vi "Main_SAIDD.vi"() -> ()   [LabVIEW 2019]
uses:
  <extravilib>/ChannelInstances/Tag-bool/Write With Abort.vi
  <extravilib>/ChannelInstances/Tag-bool/Read With Abort.vi
  <vilib>/myRIO/Common/Instrument Driver Framework/myRIO v1.0/UART/vis/myRIO v1.0 Close UART.vi
  <extravilib>/ChannelInstances/Tag-bool/Instantiate.vi
  <vilib>/Utility/error.llb/Error Cluster From Error Code.vi
  <vilib>/myRIO/Common/Instrument Driver Framework/myRIO v1.0/PWM/vis/myRIO v1.0 Write PWM.vi
  <extravilib>/ChannelInstances/Tag-bool/Endpoint.vi
  <extravilib>/ChannelInstances/Tag-bool/EndpointRead.vi
  <vilib>/myRIO/Common/Instrument Driver Framework/Utilities/vis/FPGA Ref Manager.vi
  <vilib>/myRIO/Common/Instrument Driver Framework/myRIO v1.0/myRIO v1.0 Reset FPGA.vi
  <vilib>/myRIO/Common/Instrument Driver Framework/myRIO v1.0/IRQ/vis/myRIO v1.0 IRQ Info FGV.vi
  <vilib>/myRIO/Common/Instrument Driver Framework/myRIO v1.0/IRQ/vis/myRIO v1.0 Timer IRQ Info FGV.vi
  <vilib>/myRIO/Common/Instrument Driver Framework/myRIO v1.0/IRQ/vis/myRIO v1.0 ISR Agent.vi
  <vilib>/myRIO/Instrument Drivers/Utilities/vis/Reset Index.vi
  <vilib>/myRIO/Common/Instrument Driver Framework/myRIO v1.0/Resource Manager/vis/myRIO v1.0 Block Write Resource Manager.vi
  <extravilib>/ChannelInstances/Tag-bool.lvlib
  <vilib>/myRIO/Instrument Drivers/Onboard IO/DIO/DIO.lvlib
  <vilib>/myRIO/Instrument Drivers/Onboard IO/PWM/PWM.lvlib
  <vilib>/myRIO/Instrument Drivers/Utilities/Utilities.lvlib
panel:
  out "Distance [cm]":dbl
  in  "Antal iterationer pr. stepper":i32=800
  in  "Stop":bool
  out "Measured current":dbl
  out "Ammeter measurement":dbl(graph)
  out "Duty Cycle":dbl
  out "Mean 200":dbl format="%0.2f"
  out "Battery left (%)":dbl
  in  "Drill - Frequency [Hz]":dbl=200.0
  in  "Stepper frekvens ned":dbl=120.0
  in  "Ingen modstand ned upper threshold":dbl=2750.0
  out "ALL TOP":bool
  out "ALL BOTTOM":bool
  in  "Resistance - Threshold Upper":dbl=3175.0
  in  "Resistance Threshold Lower":dbl=2975.0
  out "Process":T1(ring)
  in  "State":T1(ring)
  out "Image":T2(plugin-control)
  in  "high cutoff freq: fh":dbl=900.0
  in  "Radius":dbl=0.002 format="%#_13g"
  in  "Filter?":bool=TRUE
  out "RollDetection - Alarm":bool
  out "Data output (A3 GPS)":string[](array[string])
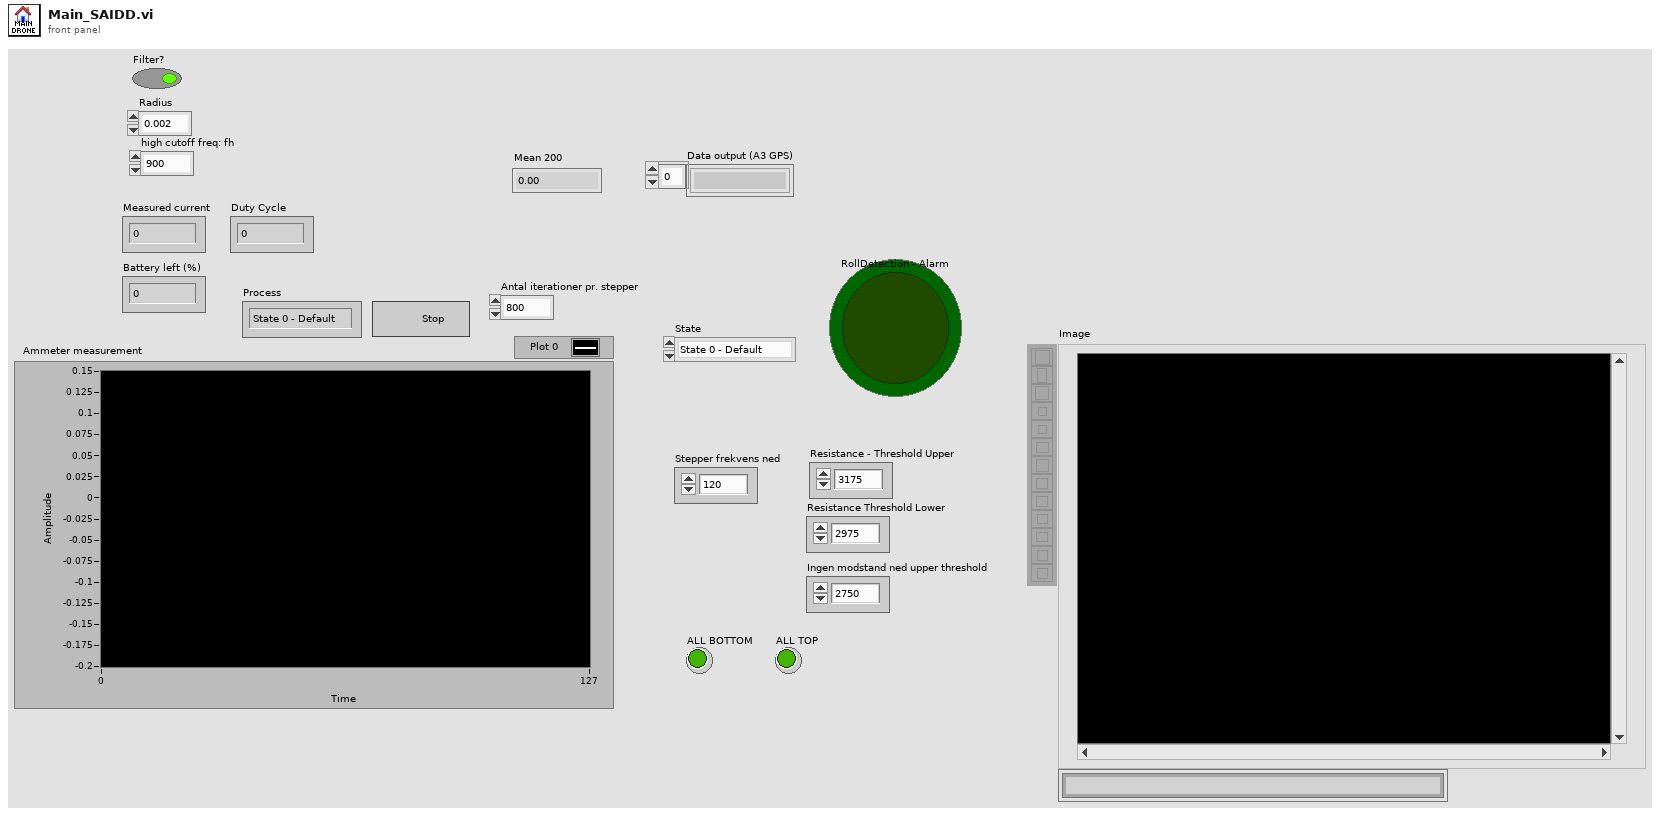
[diagram p1: front panel]
types:
  T1 = enum16{"State 0 - Default", "State 1 - Go down", "State 2 - Go up", "State 3 - Triangle Wobble"}
  T2 = typedef "IMAQ Image.ctl" = refnum<image>
  T3 = typedef "DIO.lvlib/DIO Reference.ctl" = cluster{"myRIO Reference":T4, "DIO Channels List":T8}
  T4 = typedef "myRIO Generic Hardware Reference.ctl" = cluster{"myRIO Model":T5, "myRIO Hardware Reference":T6}
  T5 = typedef "Hardware Version Enum.ctl" = enum16{"Unknown", "myRIO-1900", "myRIO-1950", "roboRIO", "NI ELVIS RIO CM", "ELVIS III"}
  T6 = typedef "myRIO v1.0 Reference.ctl" = cluster{"Generic FPGA Reference":T7, "Allow multiple opens":bool}
  T7 = typedef "Generic FPGA Reference.ctl" = refnum<k20>
  T8 = typedef "DIO Channels List.ctl" = T9[]
  T9 = typedef "DIO Channels Enum.ctl" = enum16{"Not Connected", "C/DIO0", "C/DIO1", "C/DIO2", "C/DIO3", "C/DIO4", "C/DIO5", "C/DIO6", "C/DIO7", "A/DIO0", "A/DIO1", "A/DIO2", "A/DIO3", "A/DIO4", "A/DIO5", "A/DIO6", "A/DIO7", "A/DIO8", "A/DIO9", "A/DIO10", "A/DIO11", "A/DIO12", "A/DIO13", "A/DIO14", "A/DIO15", "A/DIO16", "A/DIO17", "A/DIO18", "A/DIO19", "B/DIO0", "B/DIO1", "B/DIO2", "B/DIO3", "B/DIO4", "B/DIO5", "B/DIO6", "B/DIO7", "B/DIO8", "B/DIO9", "B/DIO10", "B/DIO11", "B/DIO12", "B/DIO13", "B/DIO14", "B/DIO15", "B/DIO16", "B/DIO17", "B/DIO18", "B/DIO19", "LED0", "LED1", "LED2", "LED3", "Button0", "DIO/DIO0", "DIO/DIO1", "DIO/DIO2", "DIO/DIO3", "DIO/DIO4", "DIO/DIO5", "DIO/DIO6", "DIO/DIO7", "DIO/DIO8", "DIO/DIO9", "SPI/CS0", "SPI/CS1", "SPI/CS2", "SPI/CS3", "LED RADIO (Green)", "LED RADIO (Red)", "LED COMM (Green)", "LED COMM (Red)", "LED MODE (Green)", "LED MODE (Red)"}
  T10 = typedef "PWM.lvlib/PWM Reference.ctl" = cluster{"myRIO Reference":T4, "PWM Channels Enum":T11, "PWM Configuration":T12}
  T11 = typedef "PWM Channels Enum.ctl" = enum16{"Not Connected", "C/PWM0", "C/PWM1", "A/PWM0", "A/PWM1", "A/PWM2", "A/PWM3", "A/PWM4", "A/PWM5", "A/PWM6", "A/PWM7", "A/PWM8", "A/PWM9", "A/PWM10", "A/PWM11", "A/PWM12", "A/PWM13", "A/PWM14", "A/PWM15", "A/PWM16", "A/PWM17", "A/PWM18", "A/PWM19", "B/PWM0", "B/PWM1", "B/PWM2", "B/PWM3", "B/PWM4", "B/PWM5", "B/PWM6", "B/PWM7", "B/PWM8", "B/PWM9", "B/PWM10", "B/PWM11", "B/PWM12", "B/PWM13", "B/PWM14", "B/PWM15", "B/PWM16", "B/PWM17", "B/PWM18", "B/PWM19", "PWM/PWM0", "PWM/PWM1", "PWM/PWM2", "PWM/PWM3", "PWM/PWM4", "PWM/PWM5", "PWM/PWM6", "PWM/PWM7", "PWM/PWM8", "PWM/PWM9"}
  T12 = typedef "PWM.lvlib/PWM Configuration.ctl" = cluster{"Frequency":dbl, "Duty Cycle":dbl}
  T13 = typedef "Accelerometer.lvlib/Accelerometer Reference.ctl" = cluster{"myRIO Reference":T4, "Accelerometer Channels List":T14, "LSB Weight":dbl}
  T14 = typedef "Accelerometer Channels List.ctl" = T15[]
  T15 = typedef "Accelerometer Channels Enum.ctl" = enum16{"Not Connected", "X-Axis", "Y-Axis", "Z-Axis"}
  T16 = typedef "AI.lvlib/AI Reference.ctl" = cluster{"myRIO Reference":T4, "AI Channels List":T17, "AI Scaling Constants List":T19}
  T17 = typedef "AI Channels List.ctl" = T18[]
  T18 = typedef "AI Channels Enum.ctl" = enum16{"Not Connected", "AudioIn/Left", "AudioIn/Right", "C/AI0", "C/AI1", "A/AI0", "A/AI1", "A/AI2", "A/AI3", "A/AI4", "A/AI5", "A/AI6", "A/AI7", "B/AI0", "B/AI1", "B/AI2", "B/AI3", "B/AI4", "B/AI5", "B/AI6", "B/AI7", "AI/AI0", "AI/AI1", "AI/AI2", "AI/AI3", "A/AI0 (DIFF)", "A/AI1 (DIFF)", "A/AI2 (DIFF)", "A/AI3 (DIFF)", "B/AI0 (DIFF)", "B/AI1 (DIFF)", "B/AI2 (DIFF)", "B/AI3 (DIFF)"}
  T19 = typedef "Analog Scaling Constants List.ctl" = T20[]
  T20 = typedef "Analog Scaling Constants.ctl" = cluster{"LSB Weight (Volts)":dbl, "Offset (Volts)":dbl, "Signed?":bool}
  T21 = typedef "SPI.lvlib/SPI Reference.ctl" = cluster{"myRIO Reference":T4, "SPI Channels Enum":T22, "SPI Configuration":T23}
  T22 = typedef "SPI Channels Enum.ctl" = enum16{"Not Connected", "A/SPI", "B/SPI", "SPI/SPI"}
  T23 = typedef "SPI.lvlib/SPI Configuration.ctl" = cluster{"Frequency [Hz]":dbl, "Clock Phase":T24, "Clock Polarity":T25, "Data Direction":T26, "Frame Length":T27}
  T24 = typedef "SPI Clock Phase.ctl" = enum8{"Leading", "Trailing"}
  T25 = typedef "SPI Clock Polarity.ctl" = enum8{"Low", "High"}
  T26 = typedef "SPI Data Direction.ctl" = enum8{"Most significant bit first", "Least significant bit first"}
  T27 = typedef "SPI Frame Length.ctl" = u8
  T28 = cluster{"B/DIO0 - Stepper Direction":T3, "B/DIO1 - Stepper1 Enable":T3, "B/DIO2 - Stepper2 Enable":T3, "B/DIO3 - Stepper3 Enable":T3, "B/DIO4 - Endstop Stepper1 Top":T3, "B/DIO11 - Endstop Stepper1 Bund":T3, "B/DIO12 - Endstop Stepper2 Top":T3, "B/DIO13 - Endstop Stepper2 Bund":T3, "B/DIO14 - Endstop Stepper3 Top":T3, "B/DIO15 - Endstop Stepper3 Bund":T3, "A/DIO0 - Cooler":T3, "A/DIO1 - Beacon drop (dio1)":T3, "A/DIO2 - Beacon drop (dio0)":T3, "A/DIO3 - QuickRelease (dio1)":T3, "A/DIO4 - QuickRelease (dio0)":T3, "A/DIO11 - LiDAR SPI CS":T3, "B/PWM0 - Stepper":T10, "B/PWM1 - Drill":T10, "A/PWM0 - Servo_Roll":T10, "A/PWM1 - Servo_Yaw":T10, "Acc. X-axis":T13, "Acc. Y-axis":T13, "B/AI0 - Beacon Drop S1 - F3":T16, "A/AI1 - Stepper Dir S3 - F4":T16, "B/AI2 - Stepper Throttle S4 - F5":T16, "B/AI3 - Drill Throttle S6 - F6":T16, "B/AI0 - Drop Drill S8 - F8":T16, "A/AI1 - Beacon Wiper":T16, "A/AI2 - QuickRelease Wiper":T16, "A/AI3 - Drill Current":T16, "A/SPI - LiDAR":T21, "B/UART - XBee":refnum<visa-resource-name>, "A/UART - A3 GPS":refnum<visa-resource-name>, "RIO Flashing LEDs":T3}
  T29 = typedef "Tag-bool.lvlib/))Channel.ctl" = refnum<queue>
  T30 = typedef "IMAQdx.ctl" = refnum<k21>
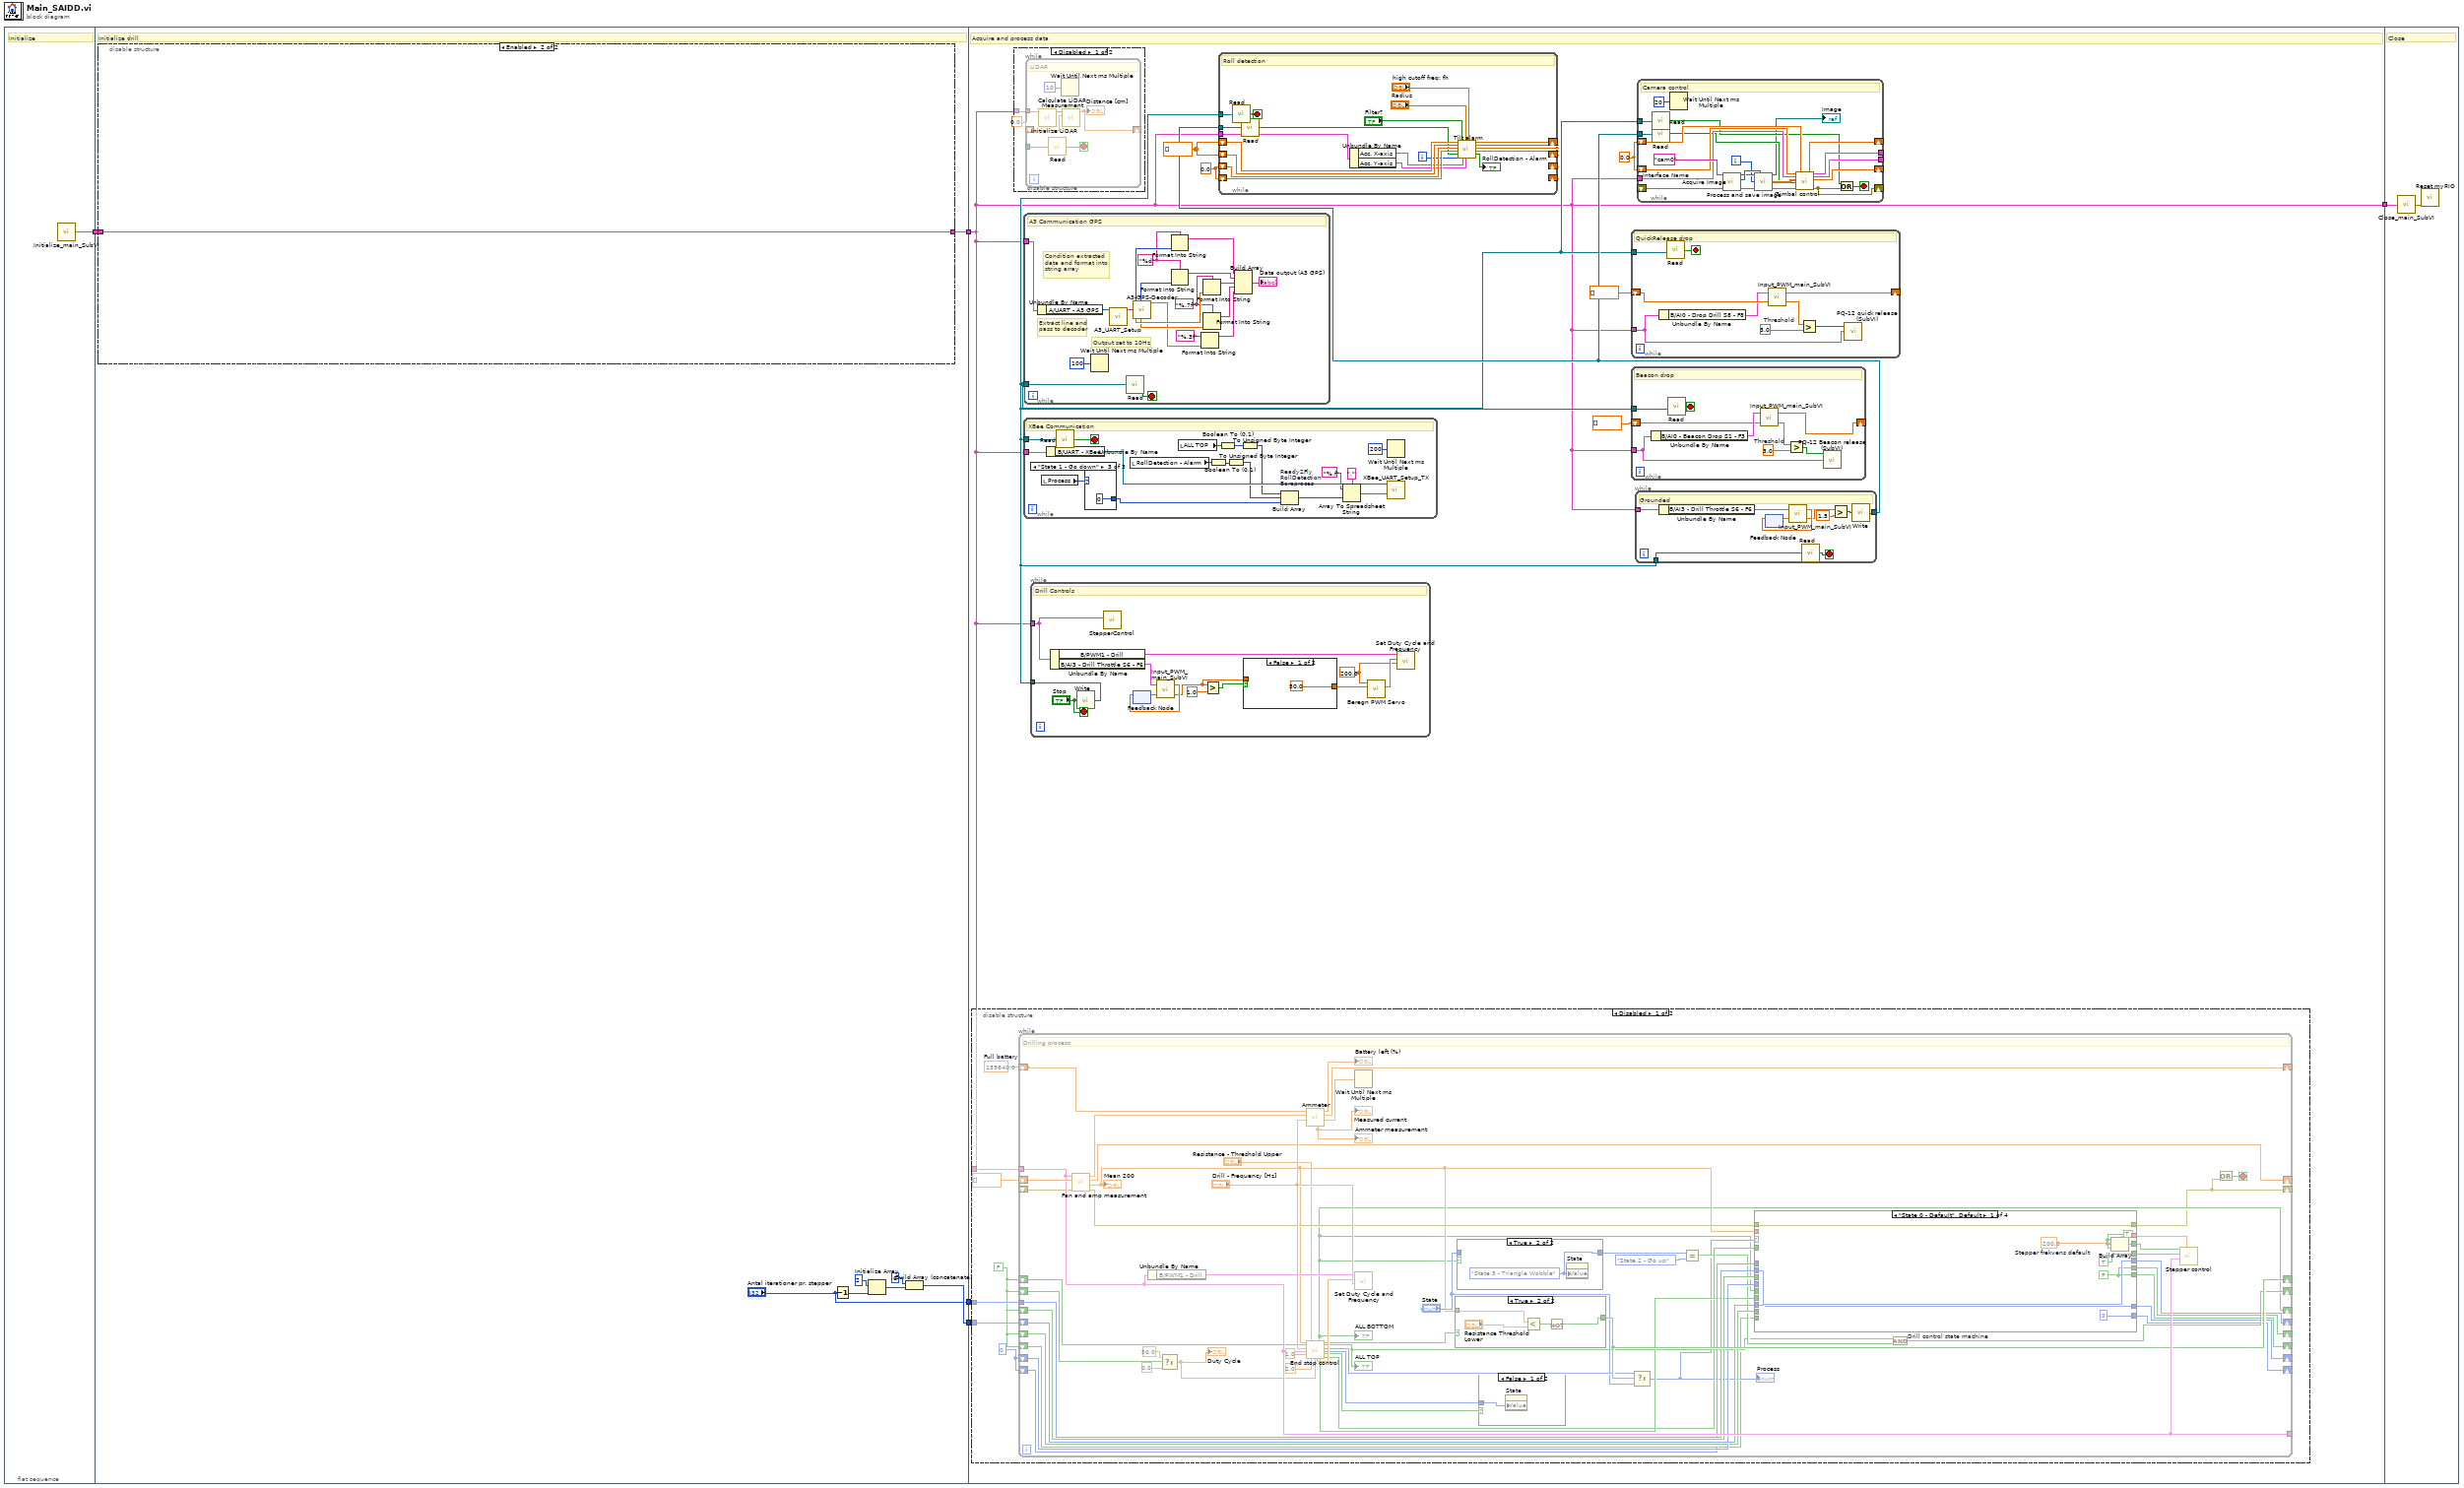
[diagram p0: block diagram]
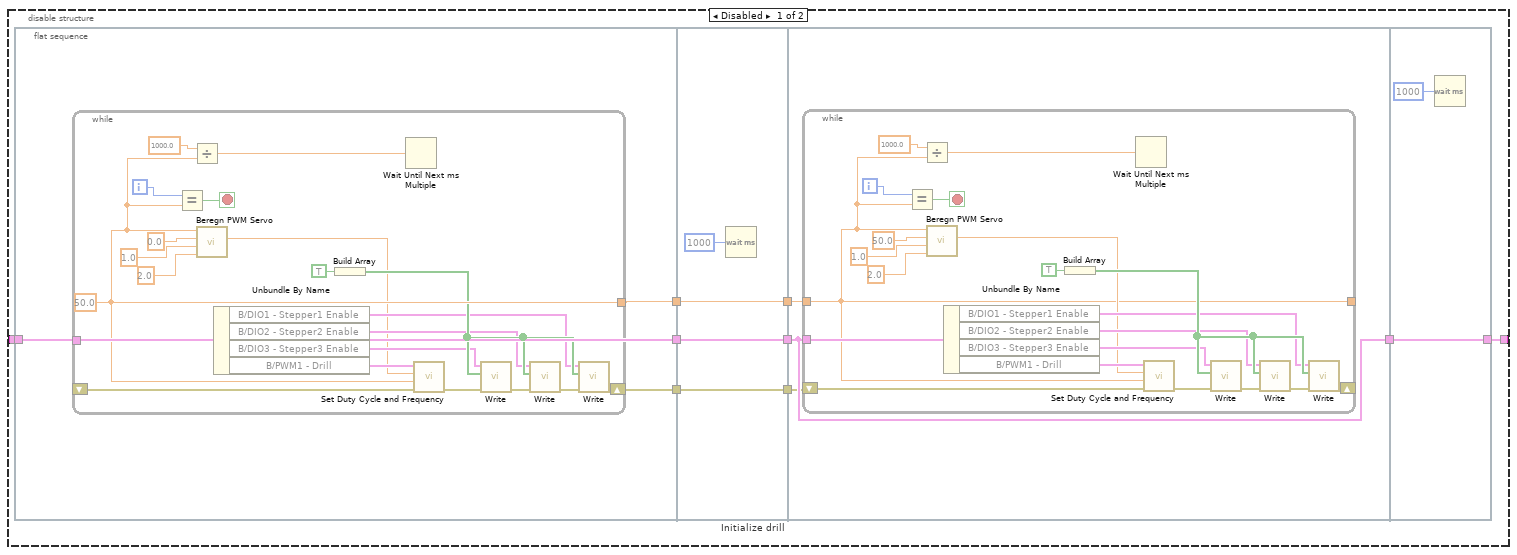
[diagram p2: hidden frame]
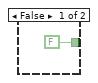
[diagram p5: hidden frame]
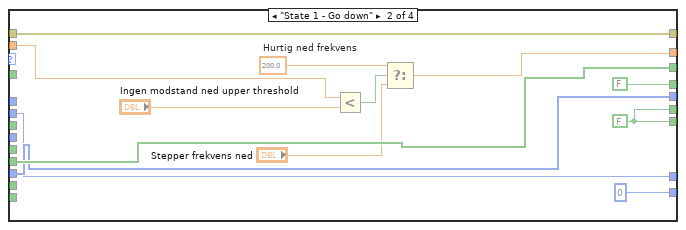
[diagram p6: hidden frame]
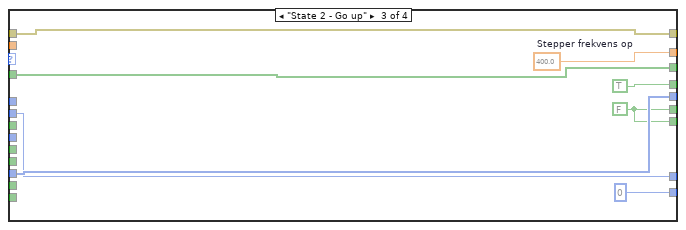
[diagram p7: hidden frame]
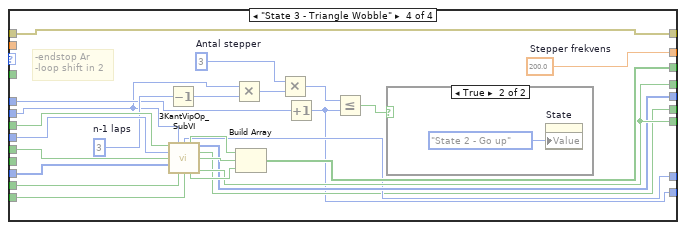
[diagram p8: hidden frame]
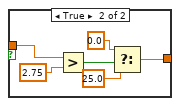
[diagram p11: hidden frame]
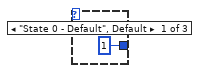
[diagram p13: hidden frame]
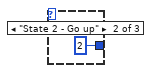
[diagram p14: hidden frame]
diagram:
  n1 = flat-sequence {
    tunnel: [w6] -> w4
    tunnel: w4 -> [w14]
    tunnel: [w13] -> w3
    tunnel: ["Antal iterationer pr. stepper"] -> w2
    tunnel: [w8] -> w1
    tunnel: w3 -> [w79]
    tunnel: [w79] -> w5
    tunnel: w2 -> [w83]
    tunnel: w1 -> [w82]
    tunnel: w5 -> [w357]
    frame #0 {
      # "Initialize"
      n2 = call "Initialize_main_SubVI.vi"() -> ("output cluster"=w6:T28)
    }
    frame #1 {
      # "Initialize drill"
      n3 = disable-structure shown="Enabled" {
        disable-tunnel: w14 -> [w16 w78]
        disable-tunnel: [w15 w78] -> w13
        frame Disabled {
          n4 = flat-sequence "Initialize drill" {
            tunnel: w16 -> [w24]
            tunnel: [w24] -> w23
            tunnel: [w26] -> w22
            tunnel: [w25] -> w21
            tunnel: w23 -> [w51]
            tunnel: [w51] -> w20
            tunnel: [w49] -> w19
            tunnel: w22 -> [w49]
            tunnel: [w48] -> w18
            tunnel: w21 -> [w48]
            tunnel: w20 -> [w54]
            tunnel: [w54] -> w17
            tunnel: w19 -> [w53]
            tunnel: w18 -> [w52]
            tunnel: [w77] -> w15
            tunnel: w17 -> [w77]
            frame #0 {
              n5 = while {
                tunnel: [w41] -> w26
                shift-right: [w33] -> w25
                shift-left: _ -> [w44]
                tunnel: w24 -> [w38]
                i -> [w43]
                stop <- w39 stop-if-true
                w41 = 50.0 ("Frequency [Hz]")
                n6 = Equal?(x=w43, y=w41) -> (x = y?=w39:bool)
                n7 = Divide(x=1000.0, y=w41) -> (x/y=w42:dbl)
                n8 = call "Beregn PWM Servo.vi"("Max (ms puls bredde)"=2.0, "Min (ms puls bredde)"=1.0, "Duty Cycle"=0.0, "Frekvens"=w41) -> ("Output Dutycycle til PWM Servo"=w27:dbl)  [unwired: 7 in]
                n9 = Unbundle By Name(w38) -> ("B/DIO1 - Stepper1 Enable"=w28:T3, "B/DIO2 - Stepper2 Enable"=w29:T3, "B/DIO3 - Stepper3 Enable"=w30:T3, "B/PWM1 - Drill"=w32:T10)
                n10 = Build Array(TRUE) -> (w31:bool[])
                n11 = Wait Until Next ms Multiple(millisecond multiple=w42) -> ()  [unwired: 1 out]
                n12 = call <vilib>:"Set Duty Cycle and Frequency.vi"("error in (no error)"=w44, "Frequency [Hz]"=w41, "Duty Cycle"=w27, "PWM Ref In"=w32) -> ("error out"=w36:errorcluster)  [unwired: 5 in, 1 out]
                n13 = call <vilib>:"Write.vi"("error in (no error)"=w36, "Values"=w31, "DIO Ref In"=w30) -> ("error out"=w35:errorcluster)  [unwired: 6 in, 1 out]
                n14 = call <vilib>:"Write.vi"("error in (no error)"=w35, "Values"=w31, "DIO Ref In"=w29) -> ("error out"=w34:errorcluster)  [unwired: 6 in, 1 out]
                n15 = call <vilib>:"Write.vi"("error in (no error)"=w34, "Values"=w31, "DIO Ref In"=w28) -> ("error out"=w33:errorcluster)  [unwired: 6 in, 1 out]
              }
            }
            frame #1 {
              n16 = Wait (ms)(milliseconds to wait=u32 1000) -> ()  [unwired: 1 out]
            }
            frame #2 {
              n17 = while {
                tunnel: [w55] -> _
                shift-right: [w62] -> _
                shift-left: w52 -> [w72]
                tunnel: w54 -> [w67]
                tunnel: w53 -> [w55]
                i -> [w71]
                stop <- w68 stop-if-true
                n18 = Equal?(x=w71, y=w55) -> (x = y?=w68:bool)
                n19 = Divide(x=1000.0, y=w55) -> (x/y=w70:dbl)
                n20 = call "Beregn PWM Servo.vi"("Max (ms puls bredde)"=2.0, "Min (ms puls bredde)"=1.0, "Duty Cycle"=50.0, "Frekvens"=w55) -> ("Output Dutycycle til PWM Servo"=w56:dbl)  [unwired: 7 in]
                n21 = Unbundle By Name(w67) -> ("B/DIO1 - Stepper1 Enable"=w57:T3, "B/DIO2 - Stepper2 Enable"=w58:T3, "B/DIO3 - Stepper3 Enable"=w59:T3, "B/PWM1 - Drill"=w61:T10)
                n22 = Build Array(TRUE) -> (w60:bool[])
                n23 = Wait Until Next ms Multiple(millisecond multiple=w70) -> ()  [unwired: 1 out]
                n24 = call <vilib>:"Set Duty Cycle and Frequency.vi"("error in (no error)"=w72, "Frequency [Hz]"=w55, "Duty Cycle"=w56, "PWM Ref In"=w61) -> ("error out"=w65:errorcluster)  [unwired: 5 in, 1 out]
                n25 = call <vilib>:"Write.vi"("error in (no error)"=w65, "Values"=w60, "DIO Ref In"=w59) -> ("error out"=w64:errorcluster)  [unwired: 6 in, 1 out]
                n26 = call <vilib>:"Write.vi"("error in (no error)"=w64, "Values"=w60, "DIO Ref In"=w58) -> ("error out"=w63:errorcluster)  [unwired: 6 in, 1 out]
                n27 = call <vilib>:"Write.vi"("error in (no error)"=w63, "Values"=w60, "DIO Ref In"=w57) -> ("error out"=w62:errorcluster)  [unwired: 6 in, 1 out]
              }
            }
            frame #3 {
              n28 = Wait (ms)(milliseconds to wait=u32 1000) -> ()  [unwired: 1 out]
            }
          }
        }
        frame Enabled {
        }
      }
      n29 = Decrement(x="Antal iterationer pr. stepper") -> (x-1=w12:i32)
      n30 = Initialize Array(2, w12) -> (w11:i32[])
      n31 = Build Array (concatenate)(6, w11) -> (w8:i32[])
    }
    frame #2 {
      w84 = 0.0 ("X-Stored-Shift-out")
      w81 = 0.0 ("Position 2")
      w88 = dbl[] [] ("X-Array-Shift-out")
      # "Acquire and process data"
      n32 = disable-structure shown="Disabled" {
        disable-tunnel: w83 -> [w92 _]
        disable-tunnel: w82 -> [w91 _]
        disable-tunnel: w79 -> [w89 _]
        frame Disabled {
          w93 = 0 ("Loops shift out")
          w90 = FALSE ("t")
          w95 = 159840.0  # Full battery
          n33 = while {
            shift-right: [w98] -> _
            shift-left: _ -> [w134]
            shift-right: [w103] -> _
            shift-left: dbl[] [] -> [w148]
            shift-right: [w144] -> _
            shift-left: w95 -> [w145]
            tunnel: w89 -> [w140]
            tunnel: [w140] -> _
            shift-right: [w136] -> _
            shift-left: w90 -> [w135]
            shift-right: [w132] -> _
            shift-left: w90 -> [w131]
            shift-right: [w129] -> _
            shift-left: w90 -> [w96]
            shift-right: [w128] -> _
            shift-left: w91 -> [w127]
            tunnel: w92 -> [w121]
            shift-right: [w125] -> _
            shift-left: w93 -> [w126]
            shift-right: [w124] -> _
            shift-left: w90 -> [w123]
            shift-right: [w100] -> _
            shift-left: w90 -> [w122]
            shift-right: [w119] -> _
            shift-left: w93 -> [w120]
            stop <- w97 stop-if-true
            # "Drilling process"
            n34 = call "Fan and amp measurement.vi"("error in (no error)"=w134, "Array in"=w148, "output cluster"=w140) -> ("error out"=w141:errorcluster, "Mean out"=w102:dbl, "Array out"=w103:dbl[], "dbl Scaled Value"=w138:dbl)  [unwired: 5 in]
            "Mean 200" <- w102
            n35 = Unbundle By Name(w140) -> ("B/PWM1 - Drill"=w142:T10)
            n36 = Select(t=50.0, s=w131, f=0.0 ("upper limit")) -> (s? t:f=w99:dbl)
            "Duty Cycle" <- w99
            n37 = call "Ammeter.vi"("Bor - Frequency [Hz]"="Drill - Frequency [Hz]", "Måling ammeter"=w138, "Sum batteri shift in"=w145) -> ("Wait ud"=w137:dbl, "Sum batteri shift ud"=w144:dbl, "Batteri tilbage (%)"=→"Battery left (%)":dbl, "Målt ampere"=→"Measured current" →"Ammeter measurement":dbl)  [unwired: 5 in]
            n38 = call "End stop control.vi"("Numeric"=w102, "t"=w135, "Bor - Frequency [Hz]"="Drill - Frequency [Hz]", "output cluster"=w140, "Min (ms puls bredde)"=1.0, "Threshold Upper"="Resistance - Threshold Upper", "Max (ms puls bredde)"=2.0, "Bor - Duty Cycle"=w99) -> ("Output Dutycycle til PWM Servo"=w147:dbl, "ALL BOTTOM"=w100:bool, "Array Bottom"=w116:bool[], "Boolean 3"=w113:bool, "ALL TOP"=w101:bool, "Enum 2"=w109:T1, "Enum"=w106:T1, "Boolean"=w107:bool, "Array Top"=w115:bool[])  [unwired: 3 in]
            "ALL TOP" <- w101
            "ALL BOTTOM" <- w100
            n39 = Wait Until Next ms Multiple(millisecond multiple=w137) -> ()  [unwired: 1 out]
            n40 = call <vilib>:"Set Duty Cycle and Frequency.vi"("Frequency [Hz]"="Drill - Frequency [Hz]", "Duty Cycle"=w147, "PWM Ref In"=w142) -> ()  [unwired: 6 in, 2 out]
            n41 = case shown="True" w113 {
              tunnel: [FALSE w155] -> w136
              tunnel: w102 -> [_ w157]
              frame False {
              }
              frame True {
                n42 = Less?(x=w157, y="Resistance Threshold Lower") -> (x < y?=w156:bool)
                n43 = Not(x=w156) -> (.not. x?=w155:bool)
              }
            }
            n44 = case shown="True" w100 {
              tunnel: [w152 w153] -> w112
              tunnel: "State" -> [w152 _]
              frame False {
              }
              frame True {
                w153 = T1."State 3 - Triangle Wobble" ("Enum")
                n45 = property on="State" class="Enum (strict)"("Value"=w153) -> ()  [unwired: 2 in, 2 out]
              }
            }
            n46 = case shown="False" w107 {
              tunnel: w106 -> [w151 _]
              frame False {
                n47 = property on="State" class="Enum (strict)"("Value"=w151) -> ()  [unwired: 2 in, 2 out]
              }
              frame True {
              }
            }
            n48 = Select(t=w109, s=w136, f="State") -> (s? t:f=w105:T1)
            "Process" <- w105
            n49 = Equal?(x=w112, y=T1."State 2 - Go up" ("Enum")) -> (x = y?=w111:bool)
            n50 = case "Drill control state machine" shown="\"State 0 - Default\", Default" w105 {
              tunnel: [w165 w180 w188 w208] -> w104
              tunnel: w116 -> [_ w180 _ _]
              tunnel: w115 -> [_ _ w188 _]
              tunnel: [TRUE FALSE TRUE w207] -> w139
              tunnel: w141 -> [w164 w178 w186 w212]
              tunnel: [w164 w178 w186 w212] -> w98
              tunnel: [w163 w175 w185 w213] -> w133
              tunnel: w102 -> [_ w172 _ _]
              tunnel: [w160 w169 w182 w207] -> w129
              tunnel: w96 -> [_ _ _ w206]
              tunnel: [w162 w171 w184 w205] -> w128
              tunnel: w127 -> [w162 w171 w184 w204]
              tunnel: w121 -> [w161 w170 w183 w194]
              tunnel: w126 -> [_ _ _ w203]
              tunnel: [w161 w170 w183 w202] -> w125
              tunnel: [w160 w169 w182 w201] -> w124
              tunnel: w123 -> [_ _ _ w200]
              tunnel: w122 -> [_ _ _ w199]
              tunnel: w100 -> [_ _ _ w197]
              tunnel: w120 -> [_ _ _ w196]
              tunnel: [0 0 0 w190] -> w119
              frame "State 0 - Default", Default {
                w160 = FALSE
                w163 = 200.0  # Stepper frekvens default
                w166 = TRUE
                n51 = Build Array(w166, w166, w166) -> (w165:bool[])
              }
              frame "State 1 - Go down" {
                w169 = FALSE
                w174 = 200.0  # Hurtig ned frekvens
                n52 = Less?(x=w172, y="Ingen modstand ned upper threshold") -> (x < y?=w177:bool)
                n53 = Select(t=w174, s=w177, f="Stepper frekvens ned") -> (s? t:f=w175:dbl)
              }
              frame "State 2 - Go up" {
                w182 = FALSE
                w185 = 400.0  # Stepper frekvens op
              }
              frame "State 3 - Triangle Wobble" {
                w192 = 3  # Antal stepper
                w198 = 3  # n-1 laps
                w213 = 200.0  # Stepper frekvens
                # "-endstop Ar\n-loop shift in 2"
                n54 = Decrement(x=w198) -> (x-1=w195:i32)
                n55 = call "3KantVipOp_SubVI.vi"("Shift 1 in"=w199, "Antal iterationer pr. stepper"=w194, "Loops shift in"=w203, "BUND!"=w197, "Index step array shift in"=w204, "Shift 2 in"=w200, "Shift 3 in"=w206) -> ("Loops shift out"=w202:i32, "Enable 1"=w209:bool, "Index step array shift ud"=w205:i32[], "Shift 2 ud"=w201:bool, "Enable 2"=w210:bool, "Enable 3"=w211:bool, "Direction"=w207:bool)  [unwired: 1 in, 1 out]
                n56 = Multiply(x=w194, y=w195) -> (x*y=w193:i32)
                n57 = Build Array(w209, w210, w211) -> (w208:bool[])
                n58 = Multiply(x=w192, y=w193) -> (x*y=w191:i32)
                n59 = Increment(x=w196) -> (x+1=w190:i32)
                n60 = Less Or Equal?(x=w191, y=w190) -> (x <= y?=w189:bool)
                n61 = case shown="True" w189 {
                  frame False {
                  }
                  frame True {
                    n62 = property on="State" class="Enum (strict)"("Value"=T1."State 2 - Go up" ("Enum")) -> ()  [unwired: 2 in, 2 out]
                  }
                }
              }
            }
            n63 = And(x=w101, y=w111) -> (x .and. y?=w132:bool)
            n64 = call "Stepper control.vi"("Stepper frekvens"=w133, "output cluster"=w140, "Direction shift ud"=w139, "Array"=w104) -> ()  [unwired: 8 in]
            n65 = Or(y=w98) -> (x .or. y?=w97:bool)  [unwired: 1 in]
          }
        }
        frame Enabled {
        }
      }
      n66 = disable-structure shown="Disabled" {
        disable-tunnel: w79 -> [w235 _]
        frame Disabled {
          n67 = while {
            tunnel: [w242] -> w237
            shift-right: [w240] -> _
            shift-left: 0.0 -> [w239]
            tunnel: w235 -> [w238]
            stop <- w241 stop-if-true
            # "LiDAR"
            n68 = call "Initialize LiDAR.vi"("output cluster"=w238) -> ("unsigned byte array"=w243:u8[])  [unwired: 10 in]
            n69 = call <extravilib>:"Read.vi"("channel"=w242) -> ("element"=w241:bool)  [unwired: 1 in, 1 out]
            n70 = Wait Until Next ms Multiple(millisecond multiple=u32 10) -> ()  [unwired: 1 out]
            n71 = call "Calculate LiDAR Measurement.vi"("Old distance"=w239, "unsigned byte array"=w243) -> ("New distance"=w240:dbl)  [unwired: 9 in]
            "Distance [cm]" <- w240
          }
        }
        frame Enabled {
        }
      }
      n72 = while {
        tunnel: [w219] -> w80
        tunnel: w79 -> [w227]
        stop <- "Stop" stop-if-true
        w218 = 200.0 ("Frequency [Hz]")
        # "Drill Controls"
        n73 = Unbundle By Name(w227) -> ("B/PWM1 - Drill"=w226:T10, "B/AI3 - Drill Throttle S6 - F6"=w222:T16)
        n74 = call <vilib>:"Write.vi"("element"="Stop") -> ("channel"=w219:T29)  [unwired: 1 out]
        n75 = call "StepperControl.vi"("output cluster"=w227) -> ()  [unwired: 11 in]
        n76 = feedback #1() -> (w223:dbl[])  [unwired: 1 in]
        n77 = call "Input_PWM_main_SubVI.vi"("Shift in"=w223, "AI Ref In"=w222) -> ("Value out"=w216:dbl, "Shift out"=w225:dbl[])
        n78 = feedback-in #1(w225) -> ()
        n79 = Greater?(x=w216, y=1.0 ("x")) -> (0:w215:bool)
        n80 = case shown="False" w215 {
          tunnel: [50.0 ("f") w229] -> w217
          tunnel: w216 -> [_ w234]
          frame False {
          }
          frame True {
            n81 = Greater?(x=w234, y=2.75) -> (0:w230:bool)
            n82 = Select(t=0.0, s=w230, f=25.0) -> (s? t:f=w229:dbl)
          }
        }
        n83 = call "Beregn PWM Servo.vi"("Duty Cycle"=w217, "Frekvens"=w218) -> ("Output Dutycycle til PWM Servo"=w221:dbl)  [unwired: 9 in]
        n84 = call <vilib>:"Set Duty Cycle and Frequency.vi"("Frequency [Hz]"=w218, "Duty Cycle"=w221, "PWM Ref In"=w226) -> ()  [unwired: 6 in, 2 out]
      }
      n85 = while {
        tunnel: w80 -> [w303]
        tunnel: w79 -> [w302]
        stop <- w304 stop-if-true
        # "XBee Communication"
        n86 = local read "Process"() -> (w295:T1)
        n87 = Unbundle By Name(w302) -> ("B/UART - XBee"=w301:refnum<visa-resource-name>)
        n88 = call <extravilib>:"Read.vi"("channel"=w303) -> ("element"=w304:bool)  [unwired: 1 in, 1 out]
        n89 = case shown="\"State 1 - Go down\"" w295 {
          tunnel: [u8 1 u8 2 u8 0] -> w294
          frame "State 0 - Default", Default {
          }
          frame "State 2 - Go up" {
          }
          frame "State 1 - Go down" {
          }
        }
        n90 = local read "RollDetection - Alarm"() -> (w290:bool)
        n91 = local read "ALL TOP"() -> (w293:bool)
        n92 = Boolean To (0,1)(Boolean=w290) -> (0, 1=w289:i16)
        n93 = Boolean To (0,1)(Boolean=w293) -> (0, 1=w292:i16)
        n94 = To Unsigned Byte Integer(number=w289) -> (unsigned 8bit integer=w288:u8)
        n95 = To Unsigned Byte Integer(number=w292) -> (unsigned 8bit integer=w291:u8)
        n96 = Build Array "Ready2Fly\nRollDetection\nBoreproces"(w291, w288, w294) -> (w297:u8[])
        n97 = Array To Spreadsheet String(delimiter (Tab)=",", array=w297, 3:"%.f" ("format string")) -> (spreadsheet string=w300:string)
        n98 = call "XBee_UART_Setup_TX.vi"("Characters to Write"=w300, "VISA resource name in"=w301) -> ()  [unwired: 9 in, 1 out]
        n99 = Wait Until Next ms Multiple(millisecond multiple=u32 200) -> ()  [unwired: 1 out]
      }
      n100 = while {
        tunnel: w79 -> [w285]
        tunnel: w80 -> [w286]
        stop <- w287 stop-if-true
        w273 = "%.7f" ("format string")
        w274 = "%d" ("format string")
        # "Output set to 10Hz"
        # "Condition extracted\ndata and format into \nstring array"
        # "Extract line and\npass to decoder"
        # "A3 Communication GPS"
        n101 = Unbundle By Name(w285) -> ("A/UART - A3 GPS"=w269:refnum<visa-resource-name>)
        n102 = Wait Until Next ms Multiple(millisecond multiple=u32 100 ("milliseconds to wait")) -> ()  [unwired: 1 out]
        n103 = call "A3_UART_Setup.vi"("VISA Refnum in"=w269) -> ("read buffer"=w270:string)  [unwired: 9 in, 1 out]
        n104 = call <extravilib>:"Read.vi"("channel"=w286) -> ("element"=w287:bool)  [unwired: 1 in, 1 out]
        n105 = call "A3-GPS-Decoder.vi"("ASCII Hexidecimal String"=w270) -> ("Date (YYYYMMDD)"=w279:u32, "Time (HHMMSS)"=w278:u32, "Longitude (Deg)"=w277:dbl, "Latitude (Deg)"=w276:dbl, "AMSL (m)"=w275:sgl)  [unwired: 3 out]
        n106 = Format Into String(format string=w274, w279) -> (resulting string=w280:string)  [unwired: 2 in, 1 out]
        n107 = Format Into String(format string=w274, w278) -> (resulting string=w284:string)  [unwired: 2 in, 1 out]
        n108 = Format Into String(format string="%.3f", w275) -> (resulting string=w281:string)  [unwired: 2 in, 1 out]
        n109 = Format Into String(format string=w273, w277) -> (resulting string=w283:string)  [unwired: 2 in, 1 out]
        n110 = Format Into String(format string=w273, w276) -> (resulting string=w282:string)  [unwired: 2 in, 1 out]
        n111 = Build Array(w280, w284, w283, w282, w281) -> (→"Data output (A3 GPS)":string[])
      }
      n112 = while {
        tunnel: w80 -> [w335]
        shift-right: [w334] -> _
        shift-left: dbl[] [] ("Shift out") -> [w333]
        tunnel: w79 -> [w329]
        stop <- w336 stop-if-true
        w332 = 3.0  # Threshold
        # "QuickRelease drop"
        n113 = Unbundle By Name(w329) -> ("B/AI0 - Drop Drill S8 - F8"=w330:T16)
        n114 = call <extravilib>:"Read.vi"("channel"=w335) -> ("element"=w336:bool)  [unwired: 1 in, 1 out]
        n115 = call "Input_PWM_main_SubVI.vi"("Shift in"=w333, "AI Ref In"=w330) -> ("Value out"=w331:dbl, "Shift out"=w334:dbl[])
        n116 = Greater?(x=w331, y=w332) -> (0:w328:bool)
        n117 = call "PQ-12 quick release (SubVI).vi"("output cluster"=w329, "Extend / Retract [F/T]"=w328) -> ()  [unwired: 1 in, 1 out]
      }
      n118 = while {
        tunnel: w79 -> [w348]
        tunnel: w80 -> [w354]
        shift-right: [w352] -> _
        shift-left: dbl[] [] ("Shift out") -> [w351]
        stop <- w355 stop-if-true
        w350 = 3.0  # Threshold
        # "Beacon drop"
        n119 = Unbundle By Name(w348) -> ("B/AI0 - Beacon Drop S1 - F3"=w353:T16)
        n120 = call <extravilib>:"Read.vi"("channel"=w354) -> ("element"=w355:bool)  [unwired: 1 in, 1 out]
        n121 = call "Input_PWM_main_SubVI.vi"("Shift in"=w351, "AI Ref In"=w353) -> ("Value out"=w349:dbl, "Shift out"=w352:dbl[])
        n122 = Greater?(x=w349, y=w350) -> (0:w347:bool)
        n123 = call "PQ-12 Beacon release (SubVI).vi"("output cluster"=w348, "Extend / Retract [T/F]"=w347) -> ()  [unwired: 1 in, 1 out]
      }
      n124 = while {
        tunnel: w80 -> [w345]
        tunnel: w79 -> [w344]
        tunnel: [w343] -> w85
        stop <- w346 stop-if-true
        # "Grounded"
        n125 = Unbundle By Name(w344) -> ("B/AI3 - Drill Throttle S6 - F6"=w338:T16)
        n126 = feedback #2() -> (w340:dbl[])  [unwired: 1 in]
        n127 = call "Input_PWM_main_SubVI.vi"("Shift in"=w340, "AI Ref In"=w338) -> ("Value out"=w339:dbl, "Shift out"=w341:dbl[])
        n128 = feedback-in #2(w341) -> ()
        n129 = call <extravilib>:"Read.vi"("channel"=w345) -> ("element"=w346:bool)  [unwired: 1 in, 1 out]
        n130 = Greater?(x=w339, y=1.5 ("x")) -> (0:w337:bool)
        n131 = call <vilib>:"Write.vi"("element"=w337) -> ("channel"=w343:T29)  [unwired: 1 out]
      }
      n132 = while {
        shift-right: [w322] -> _
        shift-left: w88 -> [w327]
        shift-right: [w321] -> _
        shift-left: w88 -> [w326]
        shift-right: [w320] -> _
        shift-left: w84 -> [w325]
        shift-right: [w319] -> _
        shift-left: w84 -> [w324]
        tunnel: w80 -> [w317]
        tunnel: w85 -> [w315]
        tunnel: w79 -> [w308]
        i -> [w323]
        stop <- w316 stop-if-true
        # "Roll detection"
        n133 = call <extravilib>:"Read.vi"("channel"=w317) -> ("element"=w316:bool)  [unwired: 1 in, 1 out]
        n134 = call <extravilib>:"Read.vi"("channel"=w315) -> ("element"=w314:bool)  [unwired: 1 in, 1 out]
        n135 = Unbundle By Name(w308) -> ("Acc. X-axis"=w312:T13, "Acc. Y-axis"=w313:T13)
        n136 = call "Tilt alarm.vi"("X-Array-Shift-in"=w327, "Y-Array-Shift-in"=w326, "X-Stored-Shift-in"=w325, "Y-Stored-Shift-in"=w324, "Grounded?"=w314, "Iterations"=w323, "Filter?"="Filter?", "Accelerometer Ref X in"=w312, "Radius"="Radius", "Accelerometer Ref Y In"=w313, "high cutoff freq: fh"="high cutoff freq: fh") -> ("X-Array-Shift-out"=w322:dbl[], "Y-Array-Shift-out"=w321:dbl[], "X-Stored-Shift-out"=w320:dbl, "Y-Stored-Shift-out"=w319:dbl, "Alarm"=→"RollDetection - Alarm":bool)  [unwired: 4 in]
      }
      n137 = while {
        shift-right: [w258] -> _
        shift-left: w81 -> [w259]
        shift-right: [w260] -> _
        shift-left: w81 -> [w261]
        tunnel: w79 -> [w252]
        tunnel: [w254] -> _
        tunnel: [w253] -> _
        tunnel: w80 -> [w251]
        tunnel: w85 -> [w248]
        shift-right: [w250] -> _
        shift-left: _ -> [w262]
        i -> [w257]
        stop <- w267 stop-if-true
        w265 = "cam0"  # Interface Name
        # "Camera control"
        n138 = call <extravilib>:"Read.vi"("channel"=w251) -> ("element"=w249:bool)  [unwired: 1 in, 1 out]
        n139 = call <extravilib>:"Read.vi"("channel"=w248) -> ("element"=w247:bool)  [unwired: 1 in, 1 out]
        n140 = Wait Until Next ms Multiple(millisecond multiple=u32 20 ("milliseconds to wait")) -> ()  [unwired: 1 out]
        n141 = call "Acquire Image.vi"("error in (no error)"=w262, "Interface Name"=w265) -> ("error out"=w266:errorcluster, "New Image"=w264:T2, "Refnum out"=w263:T30)  [unwired: 7 in]
        n142 = call "Process and save image.vi"("Refnum in"=w263, "New Image"=w264, "Numeric"=w257, "error in (no error)"=w266) -> ("Refnum out"=→"Image":T2, "Particle Measurements (Pixels)"=w255:dbl[][], "error out"=w256:errorcluster)  [unwired: 8 in, 1 out]
        n143 = call "Gimbal control.vi"("Position 5"=w261, "output cluster"=w252, "Particle Measurements (Pixels)"=w255, "element"=w247, "error in (no error)"=w256, "Position 3"=w259) -> ("Position 2"=w258:dbl, "PWM Ref Out 2"=w254:T10, "PWM Ref Out"=w253:T10, "Position 4"=w260:dbl, "error out"=w250:errorcluster)  [unwired: 6 in, 3 out]
        n144 = Or(x=w249, y=w250) -> (x .or. y?=w267:bool)
      }
    }
    frame #3 {
      # "Close"
      n145 = call "Close_main_SubVI.vi"("output cluster"=w357) -> ("error constant"=w356:errorcluster)
      n146 = call <vilib>:"Reset myRIO.vi"("error in (no error)"=w356) -> ()  [unwired: 10 in, 1 out]
    }
  }
